vi "SDO_TRAJ_ABS_ODOM_EXECUTE.vi"(6 "Pass_Through_Time":dbl=-1.0 format="%33.4f", 8 "error in (no error)":errorcluster) -> (0 "error out":errorcluster)   [LabVIEW 2019]
uses:
  <vilib>/Rock Robotics/WPI/ThirdParty/JAS_Junk/TrajLib/TypeDef/POSE2D.ctl
  <vilib>/Rock Robotics/WPI/ThirdParty/JAS_Junk/TrajLib/TypeDef/TRANSLATION2D.ctl
  <vilib>/Rock Robotics/WPI/ThirdParty/JAS_Junk/TrajLib/TypeDef/ROTATION2D.ctl
  <vilib>/Rock Robotics/WPI/ThirdParty/JAS_Junk/TrajLib/Rotation2d_Plus.vi
  <vilib>/Rock Robotics/WPI/ThirdParty/JAS_Junk/TrajLib/Twist2d_Create.vi
  <vilib>/Rock Robotics/WPI/ThirdParty/JAS_Junk/TrajLib/Rotation2d_Minus.vi
  <vilib>/Rock Robotics/WPI/ThirdParty/JAS_Junk/TrajLib/Pose2d_getTranslation.vi
  <vilib>/Rock Robotics/WPI/ThirdParty/JAS_Junk/TrajLib/Pose2d_New_TRRO.vi
  <vilib>/Rock Robotics/WPI/ThirdParty/JAS_Junk/TrajLib/VI/SwerveModulePosition_Get.vi
  <vilib>/Rock Robotics/WPI/ThirdParty/JAS_Junk/TrajLib/VI/SwerveModulePosition_New.vi
  <vilib>/Rock Robotics/WPI/ThirdParty/JAS_Junk/TrajLib/Twist2d_GetAll.vi
  <vilib>/Rock Robotics/WPI/ThirdParty/JAS_Junk/TrajLib/VI/Util_GetTime_U32.vi
  <vilib>/Rock Robotics/WPI/ThirdParty/JAS_Junk/TrajLib/Rotation2d_RotateBy.vi
  <vilib>/Rock Robotics/WPI/ThirdParty/JAS_Junk/TrajLib/Rotation2d_UnaryMinus.vi
  <vilib>/Rock Robotics/WPI/ThirdParty/JAS_Junk/TrajLib/Rotation2d_CreateXY.vi
  <vilib>/Rock Robotics/WPI/ThirdParty/JAS_Junk/TrajLib/Util_CalcDist.vi
  Swerve_Drive_System/SDO_DRIVE_GLOBALS.vi
  SDO_TRAJECTORY_GLOBALS.vi
  <vilib>/Rock Robotics/WPI/ThirdParty/JAS_Junk/TrajLib/VI/SwerveKinematics_ToTwist2dX.vi
  <vilib>/Rock Robotics/WPI/ThirdParty/JAS_Junk/TrajLib/Pose2d_Exp.vi
  <vilib>/Rock Robotics/WPI/ThirdParty/JAS_Junk/TrajLib/VI/Util_GetTime_U64.vi
  <vilib>/Rock Robotics/WPI/ThirdParty/JAS_Junk/TrajLib/Trajectory_Library.lvlib
panel:
  in  "Add Vision Meas":bool
  in  "visionRobotPose":T1={"TRANSLATION"={"X"=0.0, "Y"=0.0}, "ROTATION"={"VALUE"=0.0, "COS"=1.0, "SIN"=0.0}} {"ROTATION"."SIN" format="%13.4f"; "ROTATION"."COS" format="%13.4f"; "ROTATION"."VALUE" format="%13.4f"; "TRANSLATION"."Y" format="%14.3f"; "TRANSLATION"."X" format="%14.3f"}
  in  "Vision TImeStamp_Seconds":dbl=0.02
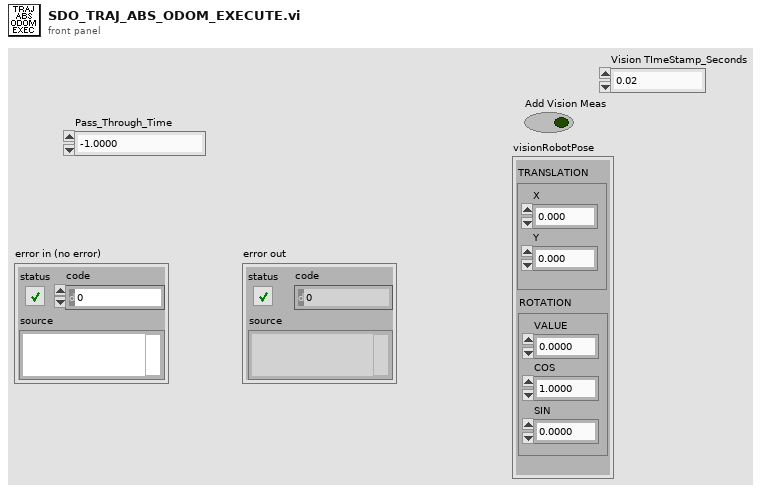
[diagram p1: front panel]
types:
  T1 = typedef "Trajectory_Library.lvlib/POSE2D.ctl" = cluster{"TRANSLATION":T2, "ROTATION":T3}
  T2 = typedef "Trajectory_Library.lvlib/TRANSLATION2D.ctl" = cluster{"X":dbl, "Y":dbl}
  T3 = typedef "Trajectory_Library.lvlib/ROTATION2D.ctl" = cluster{"VALUE":dbl, "COS":dbl, "SIN":dbl}
  T4 = typedef "Trajectory_Library.lvlib/SWERVE_DRIVE_MODULE_POSITION.ctl" = cluster{"Distance":dbl, "Angle":T3, "P":bool}
  T5 = typedef "Trajectory_Library.lvlib/SWERVE_DRIVE_KINEMATICS.ctl" = cluster{"NumModules":i32, "InverseKinematics":T6, "ForwardKinematics":T6, "Modules":T2[], "PrevCoR":T2, "SavedModuleStates":T7[]}
  T6 = typedef "NI_Matrix.lvlib/RealMatrix.ctl" = dbl[][]
  T7 = typedef "Trajectory_Library.lvlib/SWERVE_DRIVE_MODULE_STATE.ctl" = cluster{"Speed":dbl, "Angle":T3}
  T8 = typedef "Trajectory_Library.lvlib/SWERVE_DRIVE_ODOMETRY.ctl" = cluster{"POSE":T1, "GyroOffset":T3, "PreviousAngle":T3, "PrevModulePositions":T4[], "NumModules":i32}
  T9 = typedef "Trajectory_Library.lvlib/SWERVE_DRIVE_POSE_EST2_CONFIG.ctl" = cluster{"Wheel_Locations M":T2[], "Odom X std dev M":dbl, "Odom Y std dev M":dbl, "Odom Heading std dev Rad":dbl, "Vision X std dev M":dbl, "Vision Y std dev M":dbl, "Vision Heading std dev Rad":dbl}
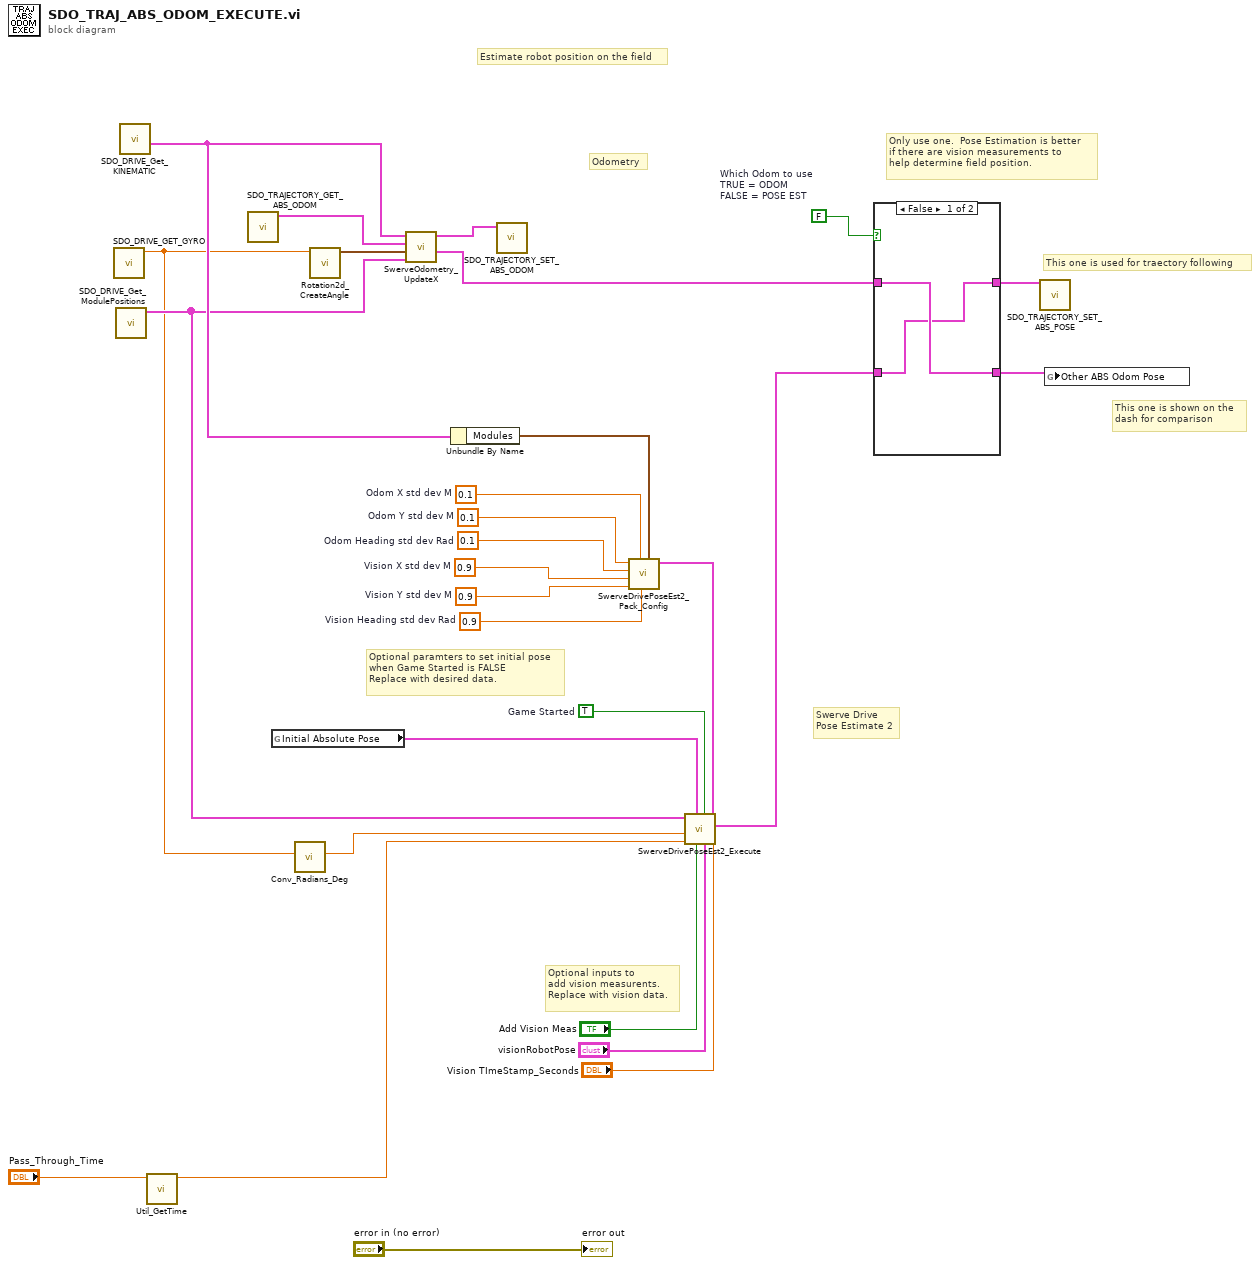
[diagram p0: block diagram]
diagram:
  w1 = FALSE  # Which Odom to use TRUE = ODOM FALSE = POSE EST
  w14 = TRUE  # Game Started
  w15 = 0.1  # Odom Y std dev M
  w16 = 0.1  # Odom Heading std dev Rad
  w17 = 0.9  # Vision X std dev M
  w18 = 0.9  # Vision Y std dev M
  w19 = 0.1  # Odom X std dev M
  w20 = 0.9  # Vision Heading std dev Rad
  # "This one is shown on the\ndash for comparison"
  # "This one is used for traectory following"
  # "Only use one.  Pose Estimation is better\nif there are vision measurements to\nhelp determine field position."
  # "Optional inputs to\nadd vision measurents.\nReplace with vision data."
  # "Optional paramters to set initial pose\nwhen Game Started is FALSE\nReplace with desired data."
  # "Swerve Drive \nPose Estimate 2"
  # "Odometry"
  # "Estimate robot position on the field"
  n1 = call "SDO_DRIVE_GET_GYRO.vi"() -> ("Gyro Heading Radians"=w7:dbl)  [unwired: 11 in]
  n2 = call "SDO_DRIVE_Get_ModulePositions.vi"() -> ("Swerve Module Positions"=w25:T4[])  [unwired: 11 in]
  n3 = call "SDO_DRIVE_Get_KINEMATIC.vi"() -> ("out SWERVE_DRIVE_KINEMATICS"=w26:T5)  [unwired: 11 in]
  n4 = call <vilib>:"Util_GetTime.vi"("Pass_Through_Time"="Pass_Through_Time") -> ("FPGA_Time_Seconds"=w27:dbl)  [unwired: 8 in, 2 out]
  n5 = call "SDO_TRAJECTORY_GET_ABS_ODOM.vi"() -> ("Absolue Odometry"=w22:T8)  [unwired: 11 in]
  n6 = global read "SDO_TRAJECTORY_GLOBALS.vi" "Initial Absolute Pose"() -> (w8:T1)
  n7 = call <vilib>:"Conv_Radians_Deg.vi"("Radians"=w7) -> ("Degrees"=w6:dbl)  [unwired: 10 in]
  n8 = call <vilib>:"Rotation2d_CreateAngle.vi"("Angle"=w7) -> ("ROTATION"=w23:T3)  [unwired: 10 in]
  n9 = call <vilib>:"SwerveOdometry_UpdateX.vi"("module Positions"=w25, "gyroAngle"=w23, "in SWERVE_DRIVE_ODOMETRY"=w22, "SWERVE_DRIVE_KINEMATICS"=w26) -> ("robot POSE"=w5:T1, "out SWERVE_DRIVE_ODOMETRY"=w21:T8)  [unwired: 5 in, 1 out]
  n10 = Unbundle By Name(w26) -> ("Modules"=w9:T2[])
  n11 = call "SDO_TRAJECTORY_SET_ABS_ODOM.vi"("Absolue Odometry"=w21) -> ()  [unwired: 11 in]
  n12 = call <vilib>:"SwerveDrivePoseEst2_Pack_Config.vi"("Wheel_Locations M"=w9, "Vision Heading std dev Rad"=w20, "Odom X std dev M"=w19, "Vision Y std dev M"=w18, "Vision X std dev M"=w17, "Odom Heading std dev Rad"=w16, "Odom Y std dev M"=w15) -> ("SwervePoseEst2Config"=w10:T9)  [unwired: 4 in]
  n13 = call <vilib>:"SwerveDrivePoseEst2_Execute.vi"("Vision TImeStamp_Seconds"="Vision TImeStamp_Seconds", "SwervePoseEst2Config"=w10, "visionRobotPose"="visionRobotPose", "Game Started"=w14, "Add Vision Meas"="Add Vision Meas", "InitialPose"=w8, "Pass Through Time"=w27, "Gyro Degrees"=w6, "Module Positions"=w25) -> ("Estimated Pose"=w3:T1)  [unwired: 1 in, 1 out]
  n14 = case shown="False" w1 {
    tunnel: w5 -> [w30 w32]
    tunnel: [w29 w32] -> w4
    tunnel: w3 -> [w29 w31]
    tunnel: [w30 w31] -> w2
    frame False {
    }
    frame True {
    }
  }
  n15 = call "SDO_TRAJECTORY_SET_ABS_POSE.vi"("Absolute Odometry Pose"=w4) -> ()  [unwired: 11 in]
  n16 = global write "SDO_TRAJECTORY_GLOBALS.vi" "Other ABS Odom Pose"(w2) -> ()
  "error out" <- "error in (no error)"
